vi "GE 5565PIORC.PIO.Read In-Place (1D SGL).vi"(5 "count (-1: all)":i32=-1, 7 "byte order (big-endian)":T1(ring), 8 "error in (no error)":errorcluster, 9 "data in":sgl[](array[numeric]), 10 "offset":u32, 11 "GE 5565PIORC in":refnum<class "GE 5565PIORC.lvclass">) -> (0 "error out":errorcluster, 1 "data out":sgl[](array[numeric]), 3 "GE 5565PIORC out":refnum<class "GE 5565PIORC.lvclass">)   [LabVIEW 2016, in "GE 5565PIORC.lvclass"]
doc: "Reads <B>count</B> elements of <B>data</B> from the specified <B>offset</B>. The number of elements transferred will be either <B>count</B> or the number of elements in <B>data</B>, whichever is smaller."
uses:
  GE 5565PIORC.lvclass
  <vilib>/Instr/_visa.llb/VISA Register Access Address Space.ctl
  GE 5565PIORC.lvclass/GE 5565PIORC.ctl
  GE 5565PIORC.VISA.Move In-Place.String (U32).vi
  GE 5565PIORC.VISA.Return Handler.vi
  <vilib>/Utility/error.llb/Error Cluster From Error Code.vi
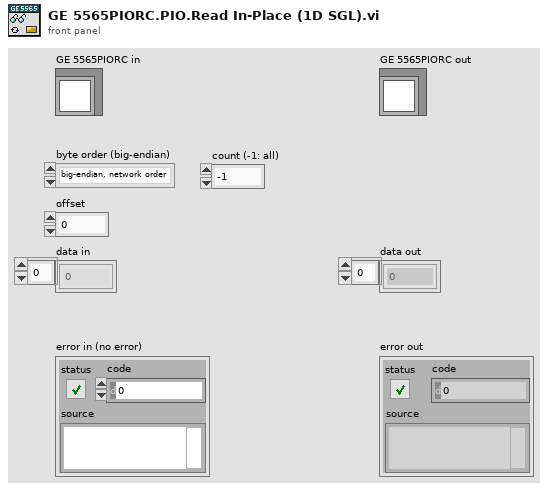
[diagram p1: front panel]
types:
  T1 = enum16{"big-endian, network order", "native, host order", "little-endian"}
  T2 = typedef "VISA Register Access Address Space.ctl" = u16
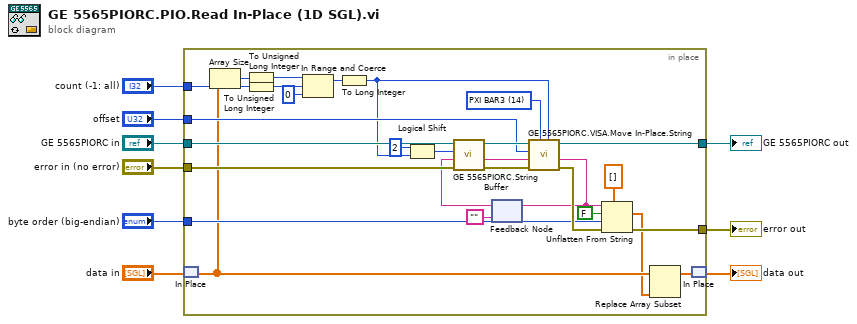
[diagram p0: block diagram]
diagram:
  n1 = in-place {
    in-place-border: "error in (no error)" -> [w27]
    in-place-border: [w37] -> w8
    in-place-border: "GE 5565PIORC in" -> [w28]
    in-place-border: "offset" -> [w18]
    in-place-border: "byte order (big-endian)" -> [w22]
    in-place-border: [w31] -> w4
    in-place-border: "count (-1: all)" -> [w20]
    w32 = T2 14 items=["VXI/VME A16"=1, "VXI/VME A24"=2, "VXI/VME A32"=3, "VXI/VME A64"=4, "PXI Memory Allocations"=9, "PXI Configuration"=10, "PXI BAR0"=11, "PXI BAR1"=12, "PXI BAR2"=13, "PXI BAR3"=14, "PXI BAR4"=15, "PXI BAR5"=16] ("address space")
    n2 = in-place-match #1("data in") -> (w17:sgl[])
    n3 = Array Size(array=w17) -> (size(s)=w34:i32)
    n4 = To Unsigned Long Integer(number=w34) -> (unsigned 32bit integer=w16:u32)
    n5 = To Unsigned Long Integer(number=w20) -> (unsigned 32bit integer=w15:u32)
    n6 = In Range and Coerce(upper limit=w16, x=w15, lower limit=u32 0) -> (coerced(x)=w19:u32)  [unwired: 1 out]
    n7 = To Long Integer(number=w19) -> (32bit integer=w13:i32)
    n8 = Logical Shift(y=i16 2, x=w13) -> (x << y=w12:i32)
    n9 = feedback #2("" ("data out")) -> (w23:string)
    n10 = call "GE 5565PIORC.String Buffer.vi"("error in (no error)"=w27, "string buffer in"=w23, "minimum size"=w12, "GE 5565PIORC in"=w28) -> ("error out"=w26:errorcluster, "string buffer out"=w25:string, "GE 5565PIORC out"=w29:refnum<class "GE 5565PIORC.lvclass">)  [unwired: 5 in]
    n11 = call-poly "GE 5565PIORC.VISA.Move In-Place.String.vi"("count (-1: all)"=w13, "address space"=w32, "error in (no error)"=w26, "data in"=w25, "offset"=w18, "GE 5565PIORC in"=w29) -> ("error out"=w30:errorcluster, "data out"=w24:string, "GE 5565PIORC out"=w31:refnum<class "GE 5565PIORC.lvclass">)  [unwired: 3 in]
    n12 = feedback-in #2(w24) -> ()
    n13 = Unflatten From String(type=sgl[] [], binary string=w24, data includes array or string size? (T)=FALSE, byte order (0:big-endian, network order)=w22, error in (no error)=w30) -> (value=w14:sgl[], error out=w37:errorcluster)  [unwired: 1 out]
    n14 = Replace Array Subset(array=w17, new element=w14) -> (w33:sgl[])  [unwired: 1 in]
    n15 = in-place-match #1(w33) -> (→"data out":sgl[])
  }
  "GE 5565PIORC out" <- w4
  "error out" <- w8
